vi "Hardware_Setting.vi"(8 "Error in":errorcluster) -> (0 "error out 2":errorcluster)   [LabVIEW 2017]
uses:
  <vilib>/Utility/error.llb/DialogType.ctl
  7b15bcbb-fc00-4973-b734-530bccfd2341.vi
  adb9f82c-1df5-4670-ad2e-9e62be5809cf.vi
  <vilib>/Utility/config.llb/NI_LVConfig.lvlib
panel:
  out "Array":string[](array[string])
  in  "Print":bool
  in  "FG CAT No.":string(combo)
  in  "Scanner Com":refnum<visa-resource-name>
  in  "PLC IP Address":string
  in  "Printer IP":string
  in  "Save Setting":bool
  in  "Close":bool
  out "error out":errorcluster
  out "Machine Name":string
  # "Resolution: 1920 x 1080 pixels"
  # "FG CAT No. + Month/year + Counter"
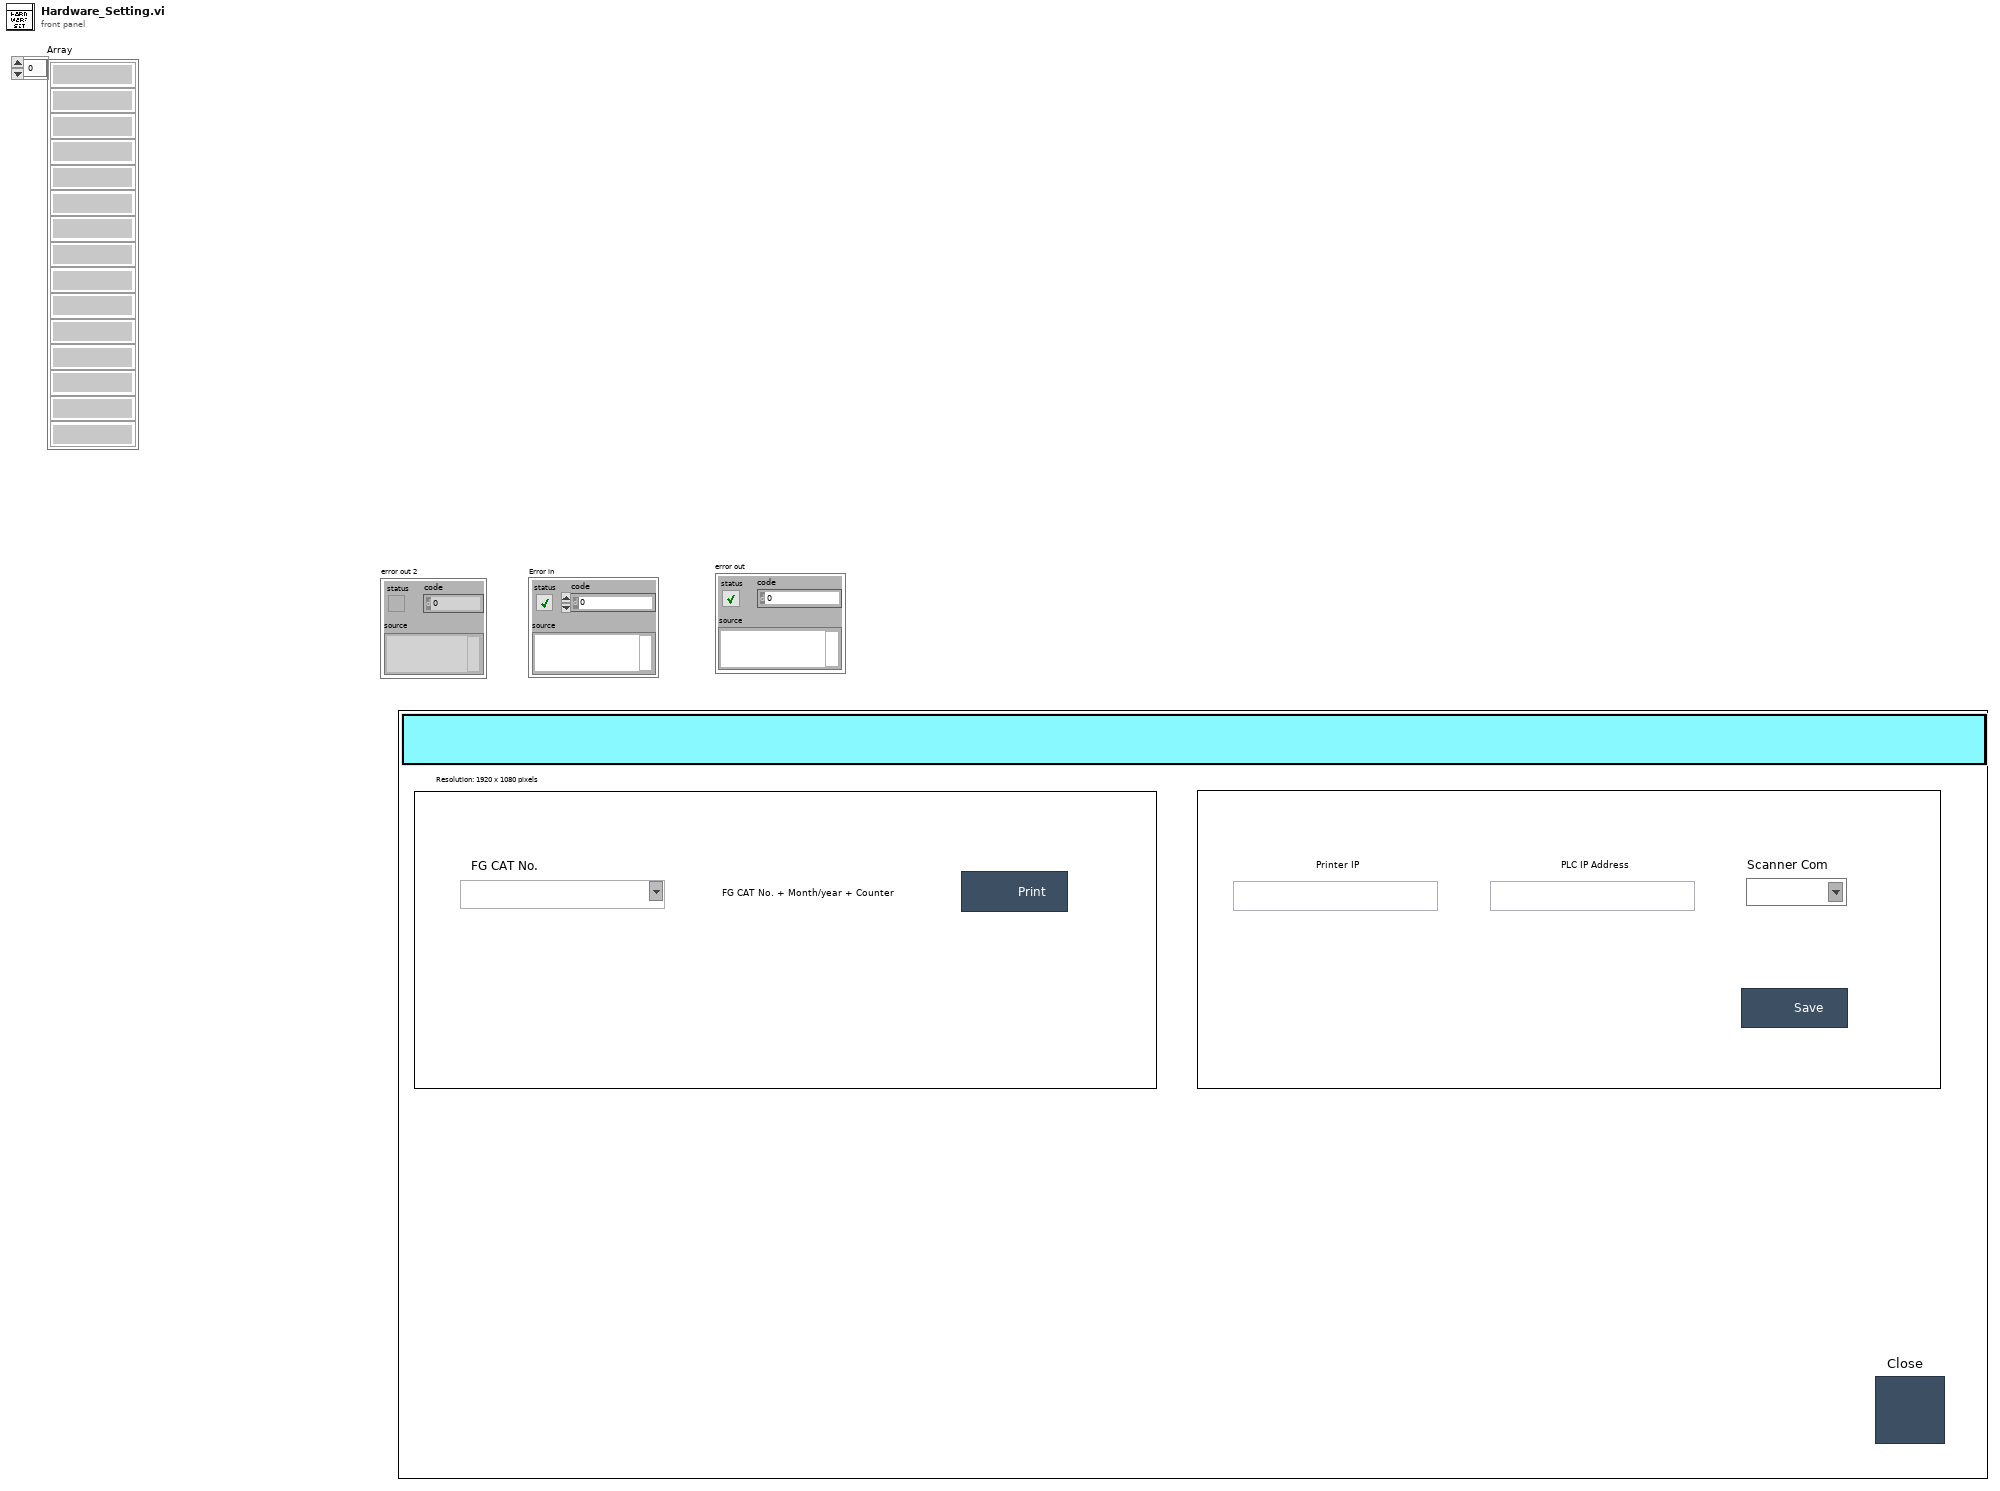
[diagram p1: front panel]
types:
  T1 = cluster{"Printer IP":string, "PLC IP Address":string, "Scanner Com":refnum<visa-resource-name>}
  T2 = enum32{"invalid app kind", "Development System", "Run Time System", "Student Edition", "Embedded LabVIEW", "Evaluation", "Custom"}
  T3 = typedef "NI_LVConfig.lvlib/Config Data RefNum.ctl" = refnum<k1>
  T4 = typedef "DialogType.ctl" = u16
  T5 = enum32{"Invalid", "Standard", "Closed", "Hidden", "Minimized", "Maximized"}
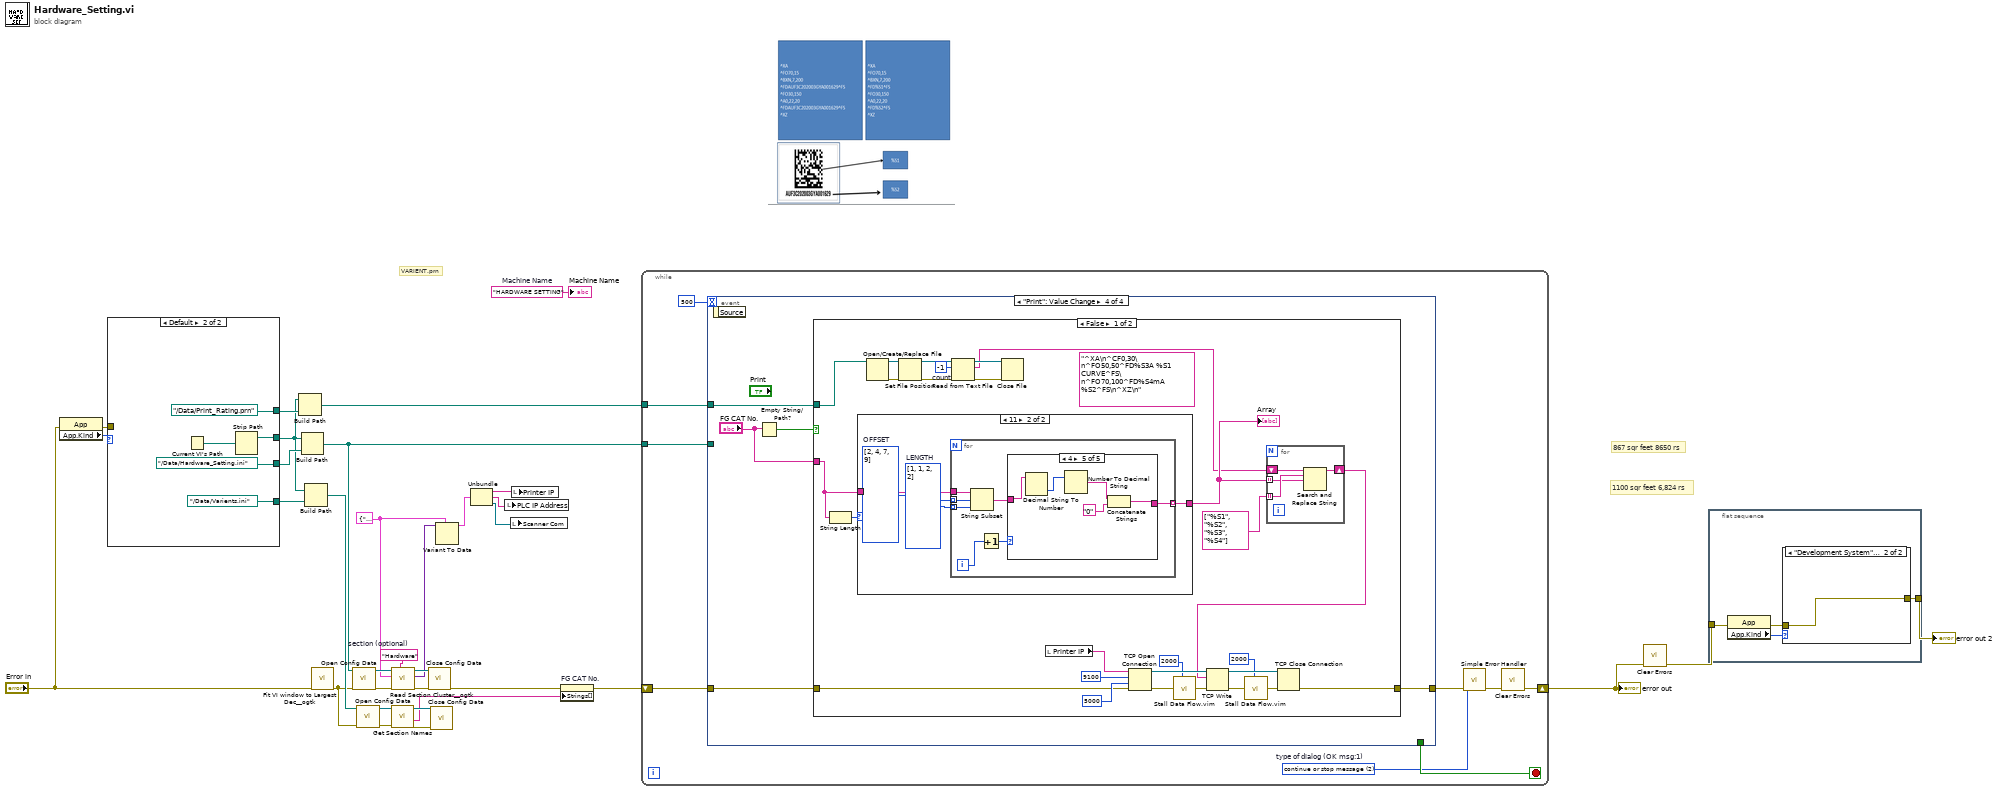
[diagram p0: block diagram]
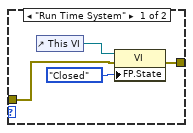
[diagram p2: hidden frame]
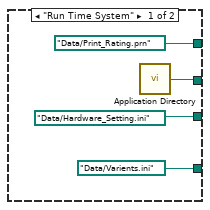
[diagram p3: hidden frame]
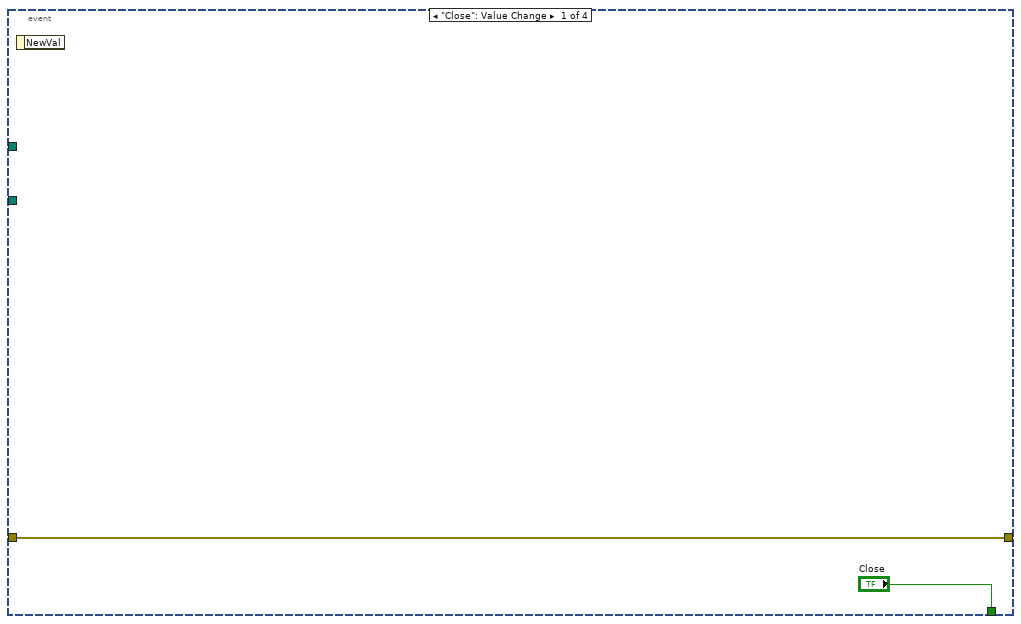
[diagram p4: hidden frame]
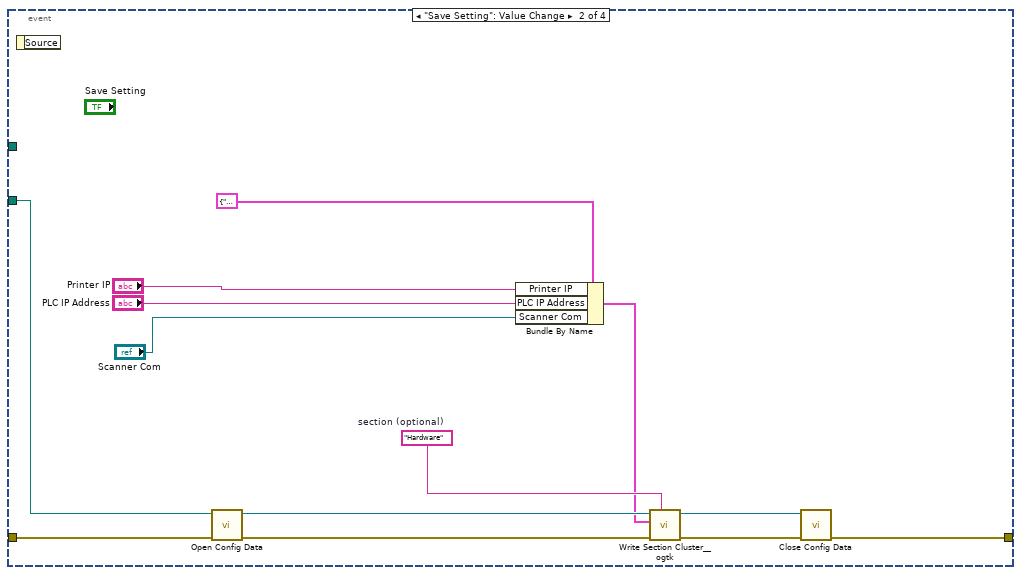
[diagram p5: hidden frame]
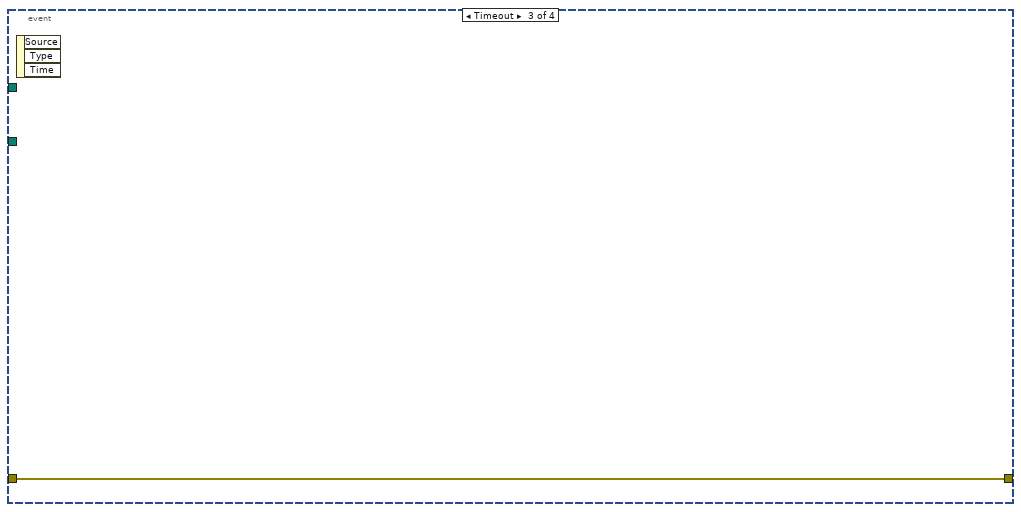
[diagram p6: hidden frame]
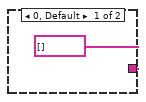
[diagram p7: hidden frame]
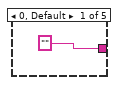
[diagram p8: hidden frame]
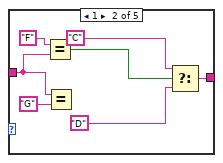
[diagram p9: hidden frame]
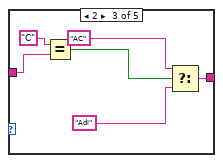
[diagram p10: hidden frame]
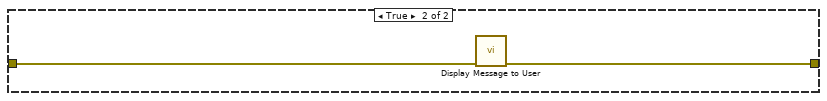
[diagram p12: hidden frame]
diagram:
  w17 = T1 {"Printer IP"="", "PLC IP Address"="", "Scanner Com"=""}
  w22 = "Hardware"  # section (optional)
  w33 = "HARDWARE SETTING"  # Machine Name
  # "VARIENT.prn"
  # "1100 sqr feet 6,824 rs"
  # "867 sqr feet 8650 rs"
  n1 = property class="App"(error in="Error in") -> (error out=w30:errorcluster, "App.Kind"=w32:T2)  [unwired: 1 in, 1 out]
  n2 = case shown="Default" w32 {
    tunnel: [path "Data/Hardware_Setting.ini" ("path") path "../Data/Hardware_Setting.ini" ("path")] -> w31
    tunnel: [w34 w40] -> w8
    tunnel: w30 -> [_ _]
    tunnel: [path "Data/Print_Rating.prn" ("path") path "../Data/Print_Rating.prn" ("path")] -> w13
    tunnel: [path "Data/Varients.ini" ("path") path "../Data/Varients.ini" ("path")] -> w9
    frame "Run Time System" {
      n3 = call <vilib>:"Application Directory.vi"() -> ("Application Directory"=w34:path)
    }
    frame Default {
      n4 = Current VI's Path() -> (path=w41:path)
      n5 = Strip Path(path=w41) -> (stripped path=w40:path)  [unwired: 1 out]
    }
  }
  n6 = Build Path(base path=w8, name or relative path=w13) -> (appended path=w12:path)
  n7 = Build Path(base path=w8, name or relative path=w31) -> (appended path=w28:path)
  n8 = Build Path(base path=w8, name or relative path=w9) -> (appended path=w7:path)
  n9 = call <userlib>:"Fit VI window to Largest Dec__ogtk.vi"("error in (no error)"="Error in") -> ("error out"=w6:errorcluster)  [unwired: 5 in, 1 out]
  n10 = call <vilib>:"Open Config Data.vi"("error in (no error)"=w6, "configuration file path"=w28) -> ("error out"=w24:errorcluster, "refnum"=w20:T3)  [unwired: 7 in, 1 out]
  n11 = call <vilib>:"Open Config Data.vi"("error in (no error)"=w6, "configuration file path"=w7) -> ("error out"=w5:errorcluster, "refnum"=w4:T3)  [unwired: 7 in, 1 out]
  n12 = call <vilib>:"Get Section Names.vi"("error in (no error)"=w5, "refnum"=w4) -> ("error out"=w2:errorcluster, "section names"=w1:string[], "refnum out"=w3:T3)  [unwired: 7 in]
  n13 = call <userlib>:"Read Section Cluster__ogtk.vi"("section (optional)"=w22, "error in (no error)"=w24, "Section Formatted Cluster Type"=w17, "refnum"=w20) -> ("error out"=w23:errorcluster, "Section Formatted Cluster"=w19:variant, "dup refnum"=w21:T3)  [unwired: 3 in, 2 out]
  n14 = call <vilib>:"Close Config Data.vi"("error in (no error)"=w23, "refnum"=w21) -> ("error out"=w11:errorcluster)  [unwired: 8 in, 1 out]
  n15 = call <vilib>:"Close Config Data.vi"("error in (no error)"=w2, "refnum"=w3) -> ()  [unwired: 8 in, 2 out]
  n16 = Variant To Data(type=w17, Variant=w19) -> (data=w18:T1)  [unwired: 1 in, 1 out]
  n17 = Unbundle(w18) -> ("Printer IP"=w16:string, "PLC IP Address"=w15:string, "Scanner Com"=w14:refnum<visa-resource-name>)
  n18 = local write "PLC IP Address"(w15) -> ()
  n19 = local write "Scanner Com"(w14) -> ()
  n20 = local write "Printer IP"(w16) -> ()
  n21 = property on="FG CAT No." class="CmbBox"(error in=w11, "Strings[]"=w1) -> (error out=w10:errorcluster)  [unwired: 1 in, 1 out]
  n22 = while {
    shift-right: [w43] -> w26
    shift-left: w10 -> [w49]
    tunnel: w28 -> [w47]
    tunnel: w12 -> [w46]
    stop <- w51 stop-if-true
    w45 = T4 2 items=["no dialog", "OK message", "continue or stop message", "OK message + warnings", "continue/stop + warnings"]  # type of dialog (OK msg:1)
    n23 = event shown="[3] \"Print\": Value Change" {
      selector: _ -> [_ _ _ _]
      dyn-events: _ -> [_ _ _ _]
      timeout: 500 -> [_ _ _ _]
      tunnel: ["Close" _ _ _] -> w51
      tunnel: [w52 w63 w67 w71] -> w50
      tunnel: w49 -> [w52 w64 w67 w72]
      tunnel: w47 -> [_ w65 _ _]
      tunnel: w46 -> [_ _ _ w68]
      event "Close": Value Change {
        n24 = event-data() -> ()  [unwired: 1 in, 1 out]
      }
      event "Save Setting": Value Change {
        w61 = "Hardware"  # section (optional)
        n25 = event-data() -> ()  [unwired: 1 in, 1 out]
        n26 = call <vilib>:"Open Config Data.vi"("error in (no error)"=w64, "configuration file path"=w65) -> ("error out"=w60:errorcluster, "refnum"=w66:T3)  [unwired: 7 in, 1 out]
        n27 = Bundle By Name(cluster=T1 {"Printer IP"="", "PLC IP Address"="", "Scanner Com"=""}, "Printer IP"="Printer IP", "PLC IP Address"="PLC IP Address", "Scanner Com"="Scanner Com") -> (w58:T1)
        n28 = call <userlib>:"Write Section Cluster__ogtk.vi"("section (optional)"=w61, "error in (no error)"=w60, "Section Formatted Cluster"=w58, "refnum"=w66) -> ("error out"=w59:errorcluster, "dup refnum"=w62:T3)  [unwired: 6 in]
        n29 = call <vilib>:"Close Config Data.vi"("error in (no error)"=w59, "refnum"=w62) -> ("error out"=w63:errorcluster)  [unwired: 8 in, 1 out]
      }
      event Timeout {
        n30 = event-data() -> ()  [unwired: 1 in, 3 out]
      }
      event "Print": Value Change {
        n31 = event-data() -> ()  [unwired: 1 in, 1 out]
        n32 = Empty String/Path?(string/path="FG CAT No.") -> (empty?=w70:bool)
        n33 = case shown="False" w70 {
          tunnel: w72 -> [w87 w137]
          tunnel: [w93 w136] -> w71
          tunnel: "FG CAT No." -> [w82 _]
          tunnel: w68 -> [w75 _]
          frame False {
            w74 = -1  # count
            (unwired) "^XA\n^CF0,30\n^FO50,50^FD%S3A %S1 CURVE^FS\n^FO70,100^FD%S4mA %S2^FS\n^XZ\n"
            n34 = String Length(string=w82) -> (length=w85:i32)
            n35 = case shown="11" w85 {
              tunnel: w82 -> [_ w104]
              tunnel: [string[] [] w101] -> w86
              frame 0, Default {
              }
              frame 11 {
                w103 = i32[] [2, 4, 7, 9]  # OFFSET
                w102 = i32[] [1, 1, 2, 2]  # LENGTH
                n36 = for {
                  tunnel: w104 -> [w111]
                  tunnel: w103 -> [w110] mode=indexing
                  tunnel: w102 -> [w109] mode=indexing
                  tunnel: [w105] -> w101 mode=indexing
                  i -> [w108]
                  n37 = String Subset(string=w111, offset (0)=w110, length (rest)=w109) -> (substring=w107:string)
                  n38 = Increment(x=w108) -> (x+1=w106:i32)
                  n39 = case shown="4" w106 {
                    tunnel: w107 -> [_ w119 w125 w126 w128]
                    tunnel: ["" w113 w120 w126 w131] -> w105
                    frame 0, Default {
                    }
                    frame 1 {
                      n40 = Equal?(x="F", y=w119) -> (x = y?=w116:bool)
                      n41 = Equal?(x=w119, y="G") -> ()  [unwired: 1 out]
                      n42 = Select(t="C", s=w116, f="D") -> (s? t:f=w113:string)
                    }
                    frame 2 {
                      n43 = Equal?(x="C", y=w125) -> (x = y?=w123:bool)
                      n44 = Select(t="AC", s=w123, f="Adi") -> (s? t:f=w120:string)
                    }
                    frame 3 {
                    }
                    frame 4 {
                      n45 = Decimal String To Number(string=w128) -> (number=w129:i32)  [unwired: 2 in, 1 out]
                      n46 = Number To Decimal String(number=w129) -> (decimal integer string=w127:string)  [unwired: 1 in]
                      n47 = Concatenate Strings(w127, "0") -> (w131:string)
                    }
                  }
                }
              }
            }
            "Array" <- w86
            n48 = Open/Create/Replace File(file path (use dialog)=w75) -> (refnum out=w80:refnum<file>, error out=w79:errorcluster)  [unwired: 5 in, 1 out]
            n49 = Set File Position(refnum=w80, error in=w79) -> (refnum out=w78:refnum<file>, error out=w81:errorcluster)  [unwired: 2 in]
            n50 = Read from Text File(file (use dialog)=w78, count=w74, error in=w81) -> (refnum out=w77:refnum<file>, text=w73:string, error out=w76:errorcluster)  [unwired: 1 in, 1 out]
            n51 = Close File(refnum=w77, error in=w76) -> ()  [unwired: 2 out]
            n52 = local read "Printer IP"() -> (w88:string)
            n53 = TCP Open Connection(address=w88, remote port or service name=9100 ("timeout ms (60000)"), timeout ms (60000)=5000, error in (no error)=w87) -> (connection ID=w98:refnum<k5>, error out=w97:errorcluster)  [unwired: 1 in]
            n54 = call "Stall Data Flow.vim"("value in"=w97, "milliseconds to wait"=u32 2000) -> ("value out"=w95:errorcluster)  [unwired: 1 out]
            n55 = for {
              tunnel: string[] ["%S1", "%S2", "%S3", "%S4"] -> [w134] mode=indexing
              shift-right: [w133] -> w83
              shift-left: w73 -> [w135]
              tunnel: w86 -> [w132] mode=indexing
              n56 = Search and Replace String(input string=w135, search string=w134, replace string=w132) -> (result string=w133:string)  [unwired: 5 in, 3 out]
            }
            n57 = TCP Write(connection ID=w98, data in=w83, error in (no error)=w95) -> (connection ID out=w96:refnum<k5>, error out=w99:errorcluster)  [unwired: 2 out]
            n58 = call "Stall Data Flow.vim"("value in"=w99, "milliseconds to wait"=u32 2000) -> ("value out"=w94:errorcluster)  [unwired: 1 out]
            n59 = TCP Close Connection(connection ID=w96, error in (no error)=w94) -> (error out=w93:errorcluster)  [unwired: 2 out]
          }
          frame True {
            n60 = call "Display Message to User"("error in (no error)"=w137) -> ("error out"=w136:errorcluster)  [unwired: 9 in, 1 out]
          }
        }
      }
    }
    n61 = call <vilib>:"Simple Error Handler.vi"("type of dialog (OK msg:1)"=w45, "error in (no error)"=w50) -> ("error out"=w44:errorcluster)  [unwired: 3 in, 4 out]
    n62 = call <vilib>:"Clear Errors.vi"("error in (no error)"=w44) -> ("error out"=w43:errorcluster)  [unwired: 5 in, 1 out]
  }
  "error out" <- w26
  n63 = call <vilib>:"Clear Errors.vi"("error in (no error)"=w26) -> ("error out"=w25:errorcluster)  [unwired: 5 in, 1 out]
  n64 = flat-sequence {
    tunnel: [w139] -> w27
    tunnel: w25 -> [w138]
    frame #0 {
      n65 = property class="App"(error in=w138) -> (error out=w140:errorcluster, "App.Kind"=w141:T2)  [unwired: 1 in, 1 out]
      n66 = case shown="\"Development System\", Default" w141 {
        tunnel: w140 -> [w143 w146]
        tunnel: [w142 w146] -> w139
        frame "Run Time System" {
          n67 = control-ref of="This VI"() -> (w145:refnum<vi>)
          n68 = property class="VI"(reference=w145, error in=w143, "FP.State"=T5."Closed" ("Front Panel Window:State")) -> (error out=w142:errorcluster)  [unwired: 1 out]
        }
        frame "Development System", Default {
        }
      }
    }
  }
  "Machine Name" <- w33
  "error out 2" <- w27
